vi "Enough_gas.vi"(1 "Table":T1[](array[typedef]) {"Row Duration (mins)" format="%#.1f"; "Row No" min=0; "Trace Gas Concentration (%)" min=0.0 format="%#.2f"; "Emission Rate (l/min)" format="%#.2f"; "Tunnel Speed" format="%#.2f"; "Start X" format="%#.2f"; "Start Y" format="%#.2f"; "Start Z" format="%#.2f"; "End X" format="%#.2f"; "End Y" format="%#.2f"; "End Z" format="%#.2f"; "Averaging time (min)" min=0.0 format="%#.1f"}) -> ()   [LabVIEW 2010]
uses:
  Traverse_cluster.ctl
  Spacing.ctl
  Controls/Multi_run_mode.ctl
  ADAM Client/Sub VIs/ADAM Controls/Client_Source_Status.ctl
  Controls/User_Specific_mode.ctl
  Globals/Extra_Commands_Global.vi
panel:
  # "X           Y            Z"
  # "Start"
  # "End"
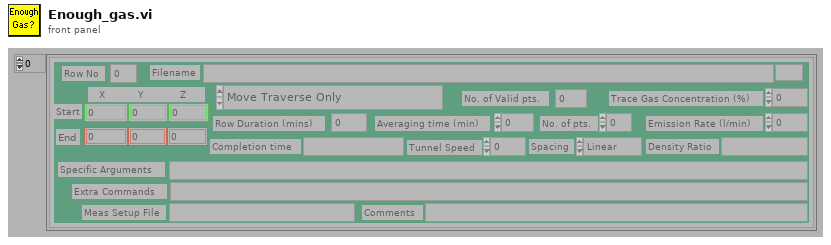
[diagram p1: front panel]
types:
  T1 = typedef "Traverse_cluster.ctl" = cluster{"Start X":dbl, "Start Y":dbl, "Start Z":dbl, "End X":dbl, "End Y":dbl, "End Z":dbl, "No. of pts.":i32, "Spacing":T2, "Filename":path, "Tunnel Speed":dbl, "Averaging time (min)":dbl, "Extra Commands":string, "Specific Arguments":string, "Emission Rate (l/min)":dbl, "Trace Gas Concentration (%)":dbl, "Density Ratio":string, "Comments":string, "Row No":i32, "Row Type Selector":T3, "Completion time":string, "Row Duration (mins)":dbl, "No. of Valid pts.":i32, "Meas Setup File":string}
  T2 = typedef "Spacing.ctl" = enum16{"Linear", "Log", "Gauss", "Specified", "N/A"}
  T3 = typedef "Multi_run_mode.ctl" = enum16{"Move Traverse Only", "Set Tunnel Speed Only", "Set Source Only", "Set Measurement Conditions", "Single Measurement", "Vertical Profile", "Lateral Profile", "Longitudinal Profile", "Explore Volume", "Multi-Axis Profile", "Auto Calibrate", "Meas Fast FID Bkgnd", "Check Beam Power", "Scanning Valve Measurement", "Run VI Named:", "Set ADAM Ch", "Wait (minutes)", "Send Message", "Synchronize With:", "Fall Back to this Row", "Turn Off Row Repeating", "Blank Row"}
  T4 = typedef "Client_Source_Status.ctl" = enum16{"Not Using", "Using", "Must Have"}
  T5 = typedef "User_Specific_mode.ctl" = enum16{"Check VI only", "Run VI"}
  T6 = typedef "Status_Cluster.ctl" = cluster{"Status":T7, "Error Type":string, "Error Description":string}
  T7 = typedef "Multi_Run_Status.ctl" = enum16{"Continue", "Jump to Next Point", "Jump to Next Row", "Jump To Fall Back", "Terminate Run"}
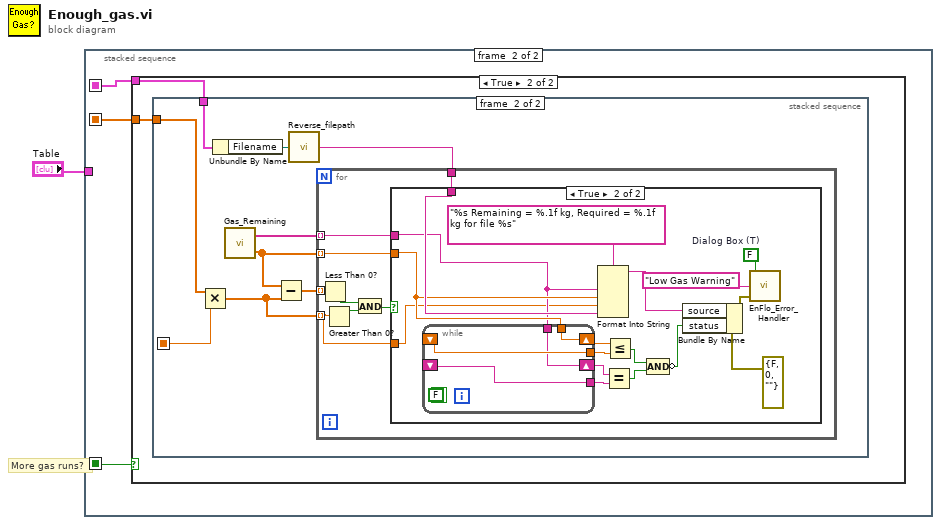
[diagram p0: block diagram]
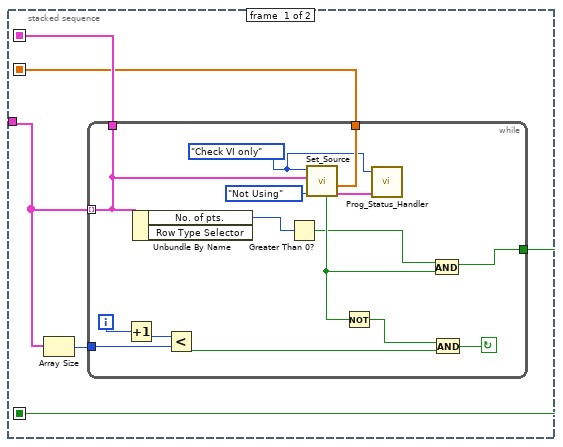
[diagram p2: hidden frame]
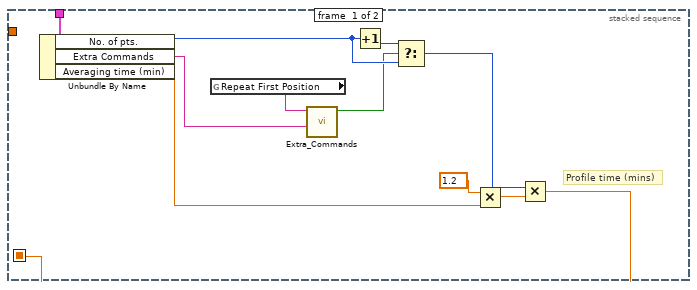
[diagram p4: hidden frame]
diagram:
  # "More gas runs?"
  n1 = stacked-sequence {
    seq-local: [w4 _] -> [_ w23]
    seq-local: [w3 _] -> [_ w22]
    seq-local: [w2 _] -> [_ w24]
    tunnel: "Table" -> [w6 _]
    frame #0 {
      n2 = Array Size(array=w6) -> (size(s)=w5:i32)
      n3 = while {
        tunnel: [w11] -> w2
        tunnel: [w16] -> w3
        tunnel: [w10] -> w4
        tunnel: w5 -> [w21]
        tunnel: w6 -> [w10] mode=indexing
        i -> [w20]
        stop <- w17 continue-if-true
        w7 = User_Specific_mode."Check VI only" ("Simulate/Run")
        n4 = Increment(x=w20) -> (x+1=w19:i32)
        n5 = Unbundle By Name(w10) -> ("No. of pts."=w14:i32)  [unwired: 1 out]
        n6 = Less?(x=w19, y=w21) -> (x < y?=w18:bool)
        n7 = Greater Than 0?(x=w14) -> (x > 0?=w12:bool)
        n8 = call "Set_Source.vi"("Source Status"=Client_Source_Status."Not Using", "Traverse line"=w10, "Simulate/Run"=w7) -> ("Status Cluster"=w8:T6, "Flowrates (kg/min)"=w16:dbl[], "Source requested?"=w13:bool)  [unwired: 1 in, 3 out]
        n9 = Not(x=w13) -> (.not. x?=w15:bool)
        n10 = call "Prog_Status_Handler.vi"("Status Cluster"=w8, "Simulate/Run"=w7) -> ()  [unwired: 2 in]
        n11 = And(x=w12, y=w13) -> (x .and. y?=w11:bool)
        n12 = And(x=w15, y=w18) -> (x .and. y?=w17:bool)
      }
    }
    frame #1 {
      n13 = case shown="True" w24 {
        tunnel: w23 -> [_ w26]
        tunnel: w22 -> [_ w25]
        frame False {
        }
        frame True {
          n14 = stacked-sequence {
            seq-local: [w31 _] -> [_ w45]
            tunnel: w26 -> [w37 w41]
            tunnel: w25 -> [_ w46]
            frame #0 {
              # "Profile time (mins)"
              n15 = Unbundle By Name(w37) -> ("No. of pts."=w33:i32, "Extra Commands"=w28:string, "Averaging time (min)"=w30:dbl)
              n16 = global read "Extra_Commands_Global.vi" "Repeat First Position"() -> (w29:string)
              n17 = call "Extra_Commands.vi"("String to Search"=w28, "Command"=w29) -> ("Command Found"=w27:bool)  [unwired: 2 in, 3 out]
              n18 = Increment(x=w33) -> (x+1=w34:i32)
              n19 = Select(t=w34, s=w27, f=w33) -> (s? t:f=w32:i32)
              n20 = Multiply(x=1.2, y=w30) -> (x*y=w35:dbl)
              n21 = Multiply(x=w32, y=w35) -> (x*y=w31:dbl)
            }
            frame #1 {
              n22 = Multiply(x=w46, y=w45) -> (x*y=w42:dbl[])
              n23 = Unbundle By Name(w41) -> ("Filename"=w39:path)
              n24 = call "Gas_Remaining.vi"() -> ("Kg Remaining"=w43:dbl[], "Gas names"=w40:string[])
              n25 = Subtract(x=w43, y=w42) -> (x-y=w44:dbl[])
              n26 = call "Reverse_filepath.vi"("Filename"=w39) -> ("Reversed Filepath"=w38:string)
              n27 = for {
                tunnel: w44 -> [w54] mode=indexing
                tunnel: w43 -> [w53] mode=indexing
                tunnel: w42 -> [w50] mode=indexing
                tunnel: w40 -> [w52] mode=indexing
                tunnel: w38 -> [w51]
                n28 = Less Than 0?(x=w54) -> (x < 0?=w48:bool)
                n29 = Greater Than 0?(x=w50) -> (x > 0?=w49:bool)
                n30 = And(x=w48, y=w49) -> (x .and. y?=w47:bool)
                n31 = case shown="True" w47 {
                  tunnel: w53 -> [_ w69]
                  tunnel: w52 -> [_ w66]
                  tunnel: w51 -> [_ w70]
                  tunnel: w50 -> [_ w61]
                  frame False {
                  }
                  frame True {
                    w59 = FALSE  # Dialog Box (T)
                    n32 = while {
                      tunnel: [w73] -> w64
                      tunnel: w66 -> [w74]
                      shift-left: _ -> [w73]
                      shift-right: [w74] -> w65
                      tunnel: [w75] -> w67
                      tunnel: w69 -> [w76]
                      shift-left: _ -> [w75]
                      shift-right: [w76] -> w68
                      stop <- FALSE continue-if-true
                    }
                    n33 = Format Into String(format string="%s Remaining = %.1f kg, Required = %.1f kg for file %s" ("Format String"), w66, w69, w61, w70) -> (resulting string=w55:string)  [unwired: 2 in, 1 out]
                    n34 = Equal?(x=w65, y=w64) -> (x = y?=w62:bool)
                    n35 = Less Or Equal?(x=w68, y=w67) -> (x <= y?=w63:bool)
                    n36 = Compound Arithmetic op=AND(w63, w62) -> (invert w57:bool)
                    n37 = Bundle By Name(cluster=errorcluster {"status"=FALSE, "code"=0, "source"=""} ("error in (no error)"), "source"=w55, "status"=w57) -> (w56:errorcluster)
                    n38 = call "EnFlo_Error_Handler.vi"("error in (no error)"=w56, "Error Type"="Low Gas Warning" ("Subject"), "Dialog Box (T)"=w59) -> ()  [unwired: 3 out]
                  }
                }
              }
            }
          }
        }
      }
    }
  }
